vi "Gen_Fault_Dataset.vi"(9 "Number of Samples Per Class":i32=5000, 11 "Dataset Folder Path":path=path "D:/Ngene/Projects_SVN/DeepLTK/Examples/2_Waveform_Processing/24_Power_Transmission_Line_Fault_Classification/Dataset/Train") -> (3 "Dataset Folder Path":path=path "D:/Ngene/Projects_SVN/DeepLTK/Examples/2_Waveform_Processing/24_Power_Transmission_Line_Fault_Classification/Dataset/Train")   [LabVIEW 2020]
uses:
  <vilib>/Utility/file.llb/Write Delimited Spreadsheet (DBL).vi
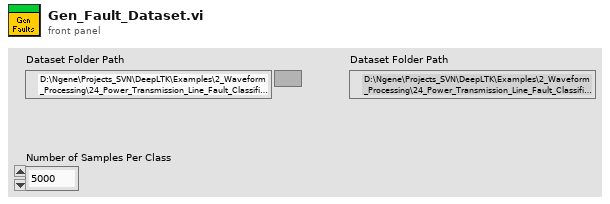
[diagram p1: front panel]
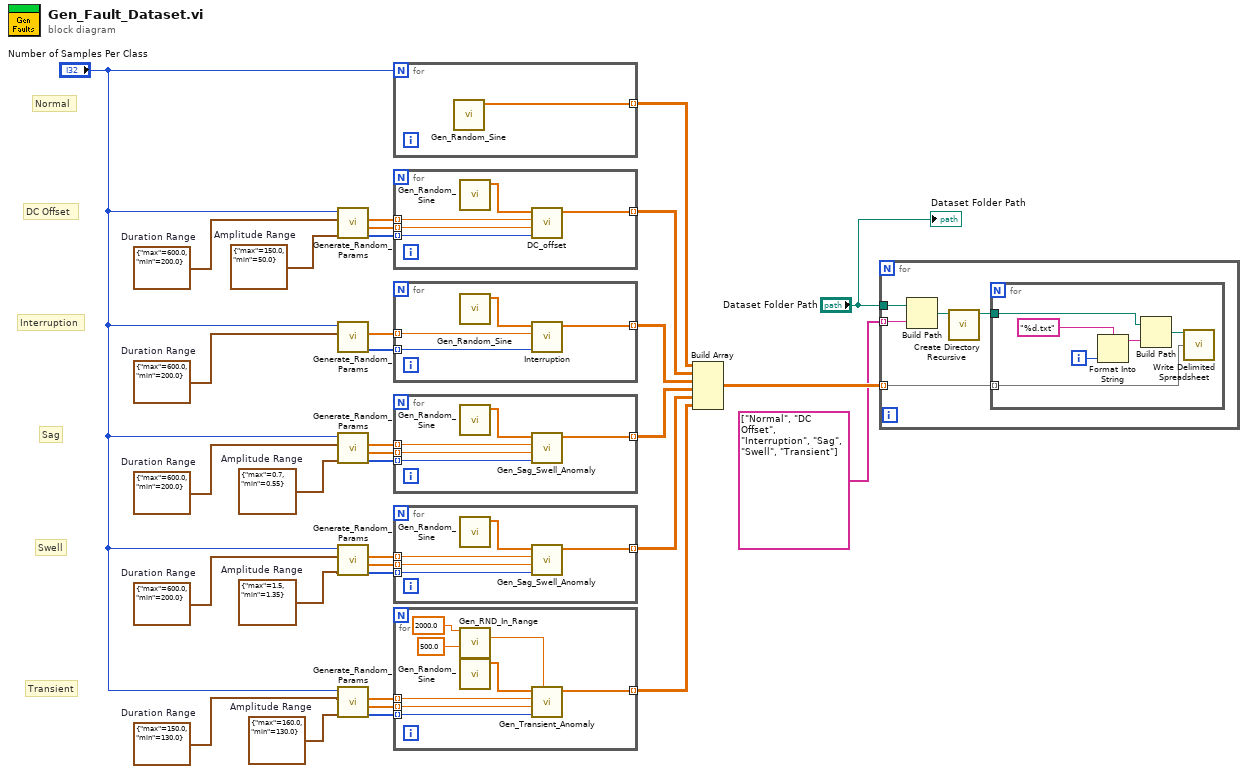
[diagram p0: block diagram]
diagram:
  w1 = cluster{"max":dbl, "min":dbl} {"max"=150.0, "min"=130.0}  # Duration Range
  w2 = cluster{"max":dbl, "min":dbl} {"max"=160.0, "min"=130.0}  # Amplitude Range
  w3 = cluster{"max":dbl, "min":dbl} {"max"=600.0, "min"=200.0}  # Duration Range
  w4 = cluster{"max":dbl, "min":dbl} {"max"=1.5, "min"=1.35}  # Amplitude Range
  w5 = cluster{"max":dbl, "min":dbl} {"max"=600.0, "min"=200.0}  # Duration Range
  w6 = cluster{"max":dbl, "min":dbl} {"max"=0.7, "min"=0.55}  # Amplitude Range
  w7 = cluster{"max":dbl, "min":dbl} {"max"=600.0, "min"=200.0}  # Duration Range
  w8 = cluster{"max":dbl, "min":dbl} {"max"=600.0, "min"=200.0}  # Duration Range
  w9 = cluster{"max":dbl, "min":dbl} {"max"=150.0, "min"=50.0}  # Amplitude Range
  # "Normal"
  # "Swell"
  # "DC Offset"
  # "Interruption"
  # "Sag"
  # "Transient"
  n1 = call "Generate_Random_Params.vi"("Amplitude Range"=w9, "Duration Range"=w8, "Samples"="Number of Samples Per Class") -> ("Duration"=w17:i32[], "Amplitude"=w18:dbl[], "Position"=w19:dbl[])  [unwired: 6 in]
  n2 = call "Generate_Random_Params.vi"("Duration Range"=w7, "Samples"="Number of Samples Per Class") -> ("Duration"=w21:i32[], "Position"=w22:dbl[])  [unwired: 7 in, 1 out]
  n3 = call "Generate_Random_Params.vi"("Amplitude Range"=w6, "Duration Range"=w5, "Samples"="Number of Samples Per Class") -> ("Duration"=w26:i32[], "Amplitude"=w25:dbl[], "Position"=w24:dbl[])  [unwired: 6 in]
  n4 = call "Generate_Random_Params.vi"("Amplitude Range"=w4, "Duration Range"=w3, "Samples"="Number of Samples Per Class") -> ("Duration"=w27:i32[], "Amplitude"=w28:dbl[], "Position"=w29:dbl[])  [unwired: 6 in]
  n5 = call "Generate_Random_Params.vi"("Amplitude Range"=w2, "Duration Range"=w1, "Samples"="Number of Samples Per Class") -> ("Duration"=w11:i32[], "Amplitude"=w10:dbl[], "Position"=w14:dbl[])  [unwired: 6 in]
  n6 = for {
    N: "Number of Samples Per Class" -> [_]
    tunnel: [w34] -> w15 mode=indexing
    n7 = call "Gen_Random_Sine.vi"() -> ("data"=w34:sgl[])  [unwired: 11 in]
  }
  n8 = for {
    tunnel: [w39] -> w16 mode=indexing
    tunnel: w19 -> [w38] mode=indexing
    tunnel: w18 -> [w37] mode=indexing
    tunnel: w17 -> [w36] mode=indexing
    n9 = call "Gen_Random_Sine.vi"() -> ("data"=w35:sgl[])  [unwired: 11 in]
    n10 = call "DC_offset.vi"("Duration"=w36, "Ampltude"=w37, "Position"=w38, "Sine"=w35) -> ("Sine+Anomaly"=w39:sgl[])  [unwired: 7 in]
  }
  n11 = for {
    tunnel: [w43] -> w20 mode=indexing
    tunnel: w22 -> [w42] mode=indexing
    tunnel: w21 -> [w41] mode=indexing
    n12 = call "Gen_Random_Sine.vi"() -> ("data"=w40:sgl[])  [unwired: 11 in]
    n13 = call "Interruption.vi"("Duration"=w41, "Position"=w42, "Sine"=w40) -> ("Sine+Anomaly"=w43:sgl[])  [unwired: 8 in]
  }
  n14 = for {
    tunnel: [w48] -> w23 mode=indexing
    tunnel: w24 -> [w47] mode=indexing
    tunnel: w25 -> [w46] mode=indexing
    tunnel: w26 -> [w45] mode=indexing
    n15 = call "Gen_Random_Sine.vi"() -> ("data"=w44:sgl[])  [unwired: 11 in]
    n16 = call "Gen_Sag_Swell_Anomaly.vi"("Duration"=w45, "Amplitude"=w46, "Position"=w47, "Sine"=w44) -> ("Sine+Anomaly"=w48:sgl[])  [unwired: 7 in]
  }
  n17 = for {
    tunnel: [w53] -> w33 mode=indexing
    tunnel: w29 -> [w52] mode=indexing
    tunnel: w28 -> [w51] mode=indexing
    tunnel: w27 -> [w50] mode=indexing
    n18 = call "Gen_Random_Sine.vi"() -> ("data"=w49:sgl[])  [unwired: 11 in]
    n19 = call "Gen_Sag_Swell_Anomaly.vi"("Duration"=w50, "Amplitude"=w51, "Position"=w52, "Sine"=w49) -> ("Sine+Anomaly"=w53:sgl[])  [unwired: 7 in]
  }
  n20 = for {
    tunnel: [w61] -> w12 mode=indexing
    tunnel: w14 -> [w60] mode=indexing
    tunnel: w11 -> [w58] mode=indexing
    tunnel: w10 -> [w54] mode=indexing
    n21 = call "Gen_RND_In_Range.vi"("Upper Bound"=2000.0 ("frequency"), "Lower Bound"=500.0 ("Variation%")) -> ("RND_In_Range"=w55:dbl)  [unwired: 13 in]
    n22 = call "Gen_Random_Sine.vi"() -> ("data"=w59:sgl[])  [unwired: 11 in]
    n23 = call "Gen_Transient_Anomaly.vi"("Frequency"=w55, "Tau"=w58, "Amplitude"=w54, "Position"=w60, "Sine"=w59) -> ("Sine+Anomaly"=w61:sgl[])  [unwired: 6 in]
  }
  n24 = Build Array(w15, w16, w20, w23, w33, w12) -> (w32:sgl[][][])
  n25 = for {
    tunnel: w32 -> [w66] mode=indexing
    tunnel: "Dataset Folder Path" -> [w65]
    tunnel: string[] ["Normal", "DC Offset", "Interruption", "Sag", "Swell", "Transient"] -> [w63] mode=indexing
    n26 = Build Path(base path=w65, name or relative path=w63) -> (appended path=w64:path)
    n27 = call <vilib>:"Create Directory Recursive.vi"("directory"=w64) -> ("directory copy"=w62:path)  [unwired: 4 in, 2 out]
    n28 = for {
      tunnel: w66 -> [w71] mode=indexing
      tunnel: w62 -> [w72]
      i -> [w68]
      n29 = Format Into String(format string="%d.txt", w68) -> (resulting string=w67:string)  [unwired: 2 in, 1 out]
      n30 = Build Path(base path=w72, name or relative path=w67) -> (appended path=w70:path)
      n31 = call-poly <vilib>:"Write Delimited Spreadsheet.vi"("file path (dialog if empty)"=w70, "1D data"=w71) -> ()  [unwired: 12 in, 2 out]
    }
  }
  "Dataset Folder Path" <- "Dataset Folder Path"
